vi "MD5Checksum pad.vi"(9 "Message String Length (bytes)":i64, 10 "Last Part of Message String":string) -> (2 "Padding":string)   [LabVIEW 2016]
doc: "This VI creates a new string that represents the padding for the message string. The sum of the lengths of the message string and the padding string (in bytes) must be a multiple of 64."
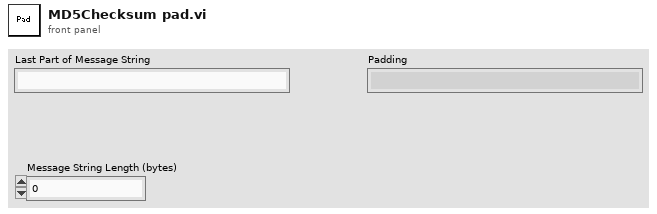
[diagram p1: front panel]
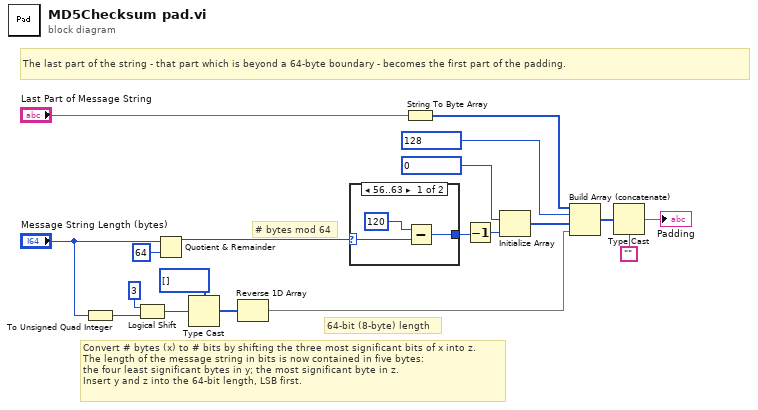
[diagram p0: block diagram]
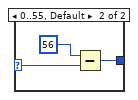
[diagram p2: hidden frame]
diagram:
  # "The last part of the string - that part which is beyond a 64-byte boundary - becomes the first part of the padding."
  # "64-bit (8-byte) length"
  # "Convert # bytes (x) to # bits by shifting the three most significant bits of x into z.\nThe length of the message string in bits is now contained in five bytes:  \nthe four least significant bytes in y; the most significant byte in z.\nInsert y and z into the 64-bit length, LSB first."
  # "# bytes mod 64"
  n1 = To Unsigned Quad Integer(1:"Message String Length (bytes)") -> (0:w5:u64)
  n2 = Logical Shift(y=i16 3, x=w5) -> (x << y=w3:u64)
  n3 = Quotient & Remainder(x="Message String Length (bytes)", y=i64 64) -> (x-y*floor(x/y)=w11:i64)  [unwired: 1 out]
  n4 = Type Cast(type=u8[] [], x=w3) -> (*(type *) &x=w2:u8[])
  n5 = Reverse 1D Array(array=w2) -> (reversed array=w1:u8[])
  n6 = case shown="56..63" w11 {
    selector: w11 -> [w21 w24]
    tunnel: [w20 w23] -> w13
    frame 56..63 {
      n7 = Subtract(x=i64 120, y=w21) -> (x-y=w20:i64)
    }
    frame 0..55, Default {
      n8 = Subtract(x=i64 56, y=w24) -> (x-y=w23:i64)
    }
  }
  n9 = String To Byte Array(string="Last Part of Message String") -> (unsigned byte array=w12:u8[])
  n10 = Decrement(x=w13) -> (x-1=w14:i64)
  n11 = Initialize Array(u8 0, w14) -> (w18:u8[])
  n12 = Build Array (concatenate)(w12, u8 128, w18, w1) -> (w15:u8[])
  n13 = Type Cast(type="", x=w15) -> (*(type *) &x=→"Padding":string)
